vi "niFPGA Rate Limiter_m.vi"   [LabVIEW 2017]
doc: "Specifies a maximum rate of change of a signal. The data type you wire to <B>input</B> determines the <B>output</B> data type."
uses:
  <vilib>/rvi/Analysis/common/FxpNativeNode/niFpgaFxpNative.xnode
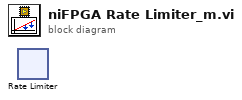
[diagram p0: block diagram]
diagram:
  n1 = xnode ("Rate Limiter")() -> ()  [unwired: 4 in, 1 out]
